vi "Name Value Pairs to JSON.vi"(9 "Message":string[][](array[string])) -> (2 "JSON string":string)   [LabVIEW 2018]
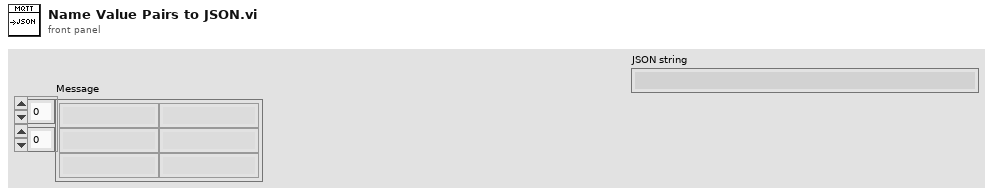
[diagram p1: front panel]
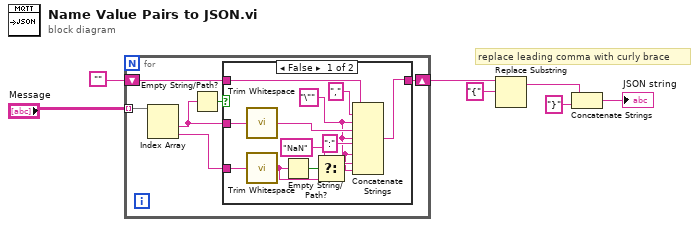
[diagram p0: block diagram]
diagram:
  # "replace leading comma with curly brace"
  n1 = for {
    tunnel: "Message" -> [w13] mode=indexing
    shift-right: [w8] -> w6
    shift-left: "" -> [w9]
    n2 = Index Array(array=w13) -> (element #1=w11:string, element #2=w10:string)  [unwired: 2 in]
    n3 = Empty String/Path?(string/path=w11) -> (empty?=w12:bool)
    n4 = case shown="False" w12 {
      tunnel: w11 -> [w25 _]
      tunnel: w10 -> [w24 _]
      tunnel: w9 -> [w20 w26]
      tunnel: [w19 w26] -> w8
      frame False {
        w14 = "\"" ("string")
        n5 = call <vilib>:"Trim Whitespace.vi"("string"=w25) -> ("trimmed string"=w17:string)  [unwired: 1 in]
        n6 = call <vilib>:"Trim Whitespace.vi"("string"=w24) -> ("trimmed string"=w22:string)  [unwired: 1 in]
        n7 = Empty String/Path?(string/path=w22) -> (empty?=w23:bool)
        n8 = Select(t="NaN", s=w23, f=w22) -> (s? t:f=w15:string)
        n9 = Concatenate Strings(w20, "," ("string"), w14, w17, w14, ":" ("string"), w14, w15, w14) -> (w19:string)
      }
      frame True {
      }
    }
  }
  n10 = Replace Substring(4:"{" ("substring (\"\")"), 5:w6) -> (1:w5:string)  [unwired: 2 in, 1 out]
  n11 = Concatenate Strings(w5, "}" ("string")) -> (→"JSON string":string)
